vi "libssh2_session_disconnect_ex.vi"(7 "lang":string, 8 "error in (no error)":errorcluster, 9 "description":string, 10 "reason":i32, 11 "Session":T1) -> (0 "error out":errorcluster, 3 "return value":i32)   [LabVIEW 2013, in "libssh2.lvlib"]
uses:
  libssh2.lvlib
  Session Refnum.ctl
  libssh2.dll
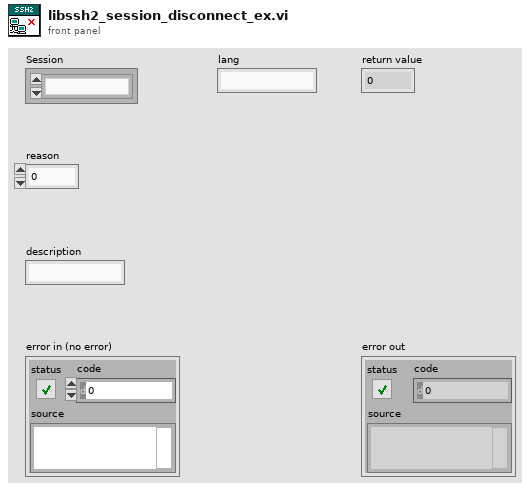
[diagram p1: front panel]
types:
  T1 = typedef "libssh2.lvlib/Session Refnum.ctl" = refnum<k1>
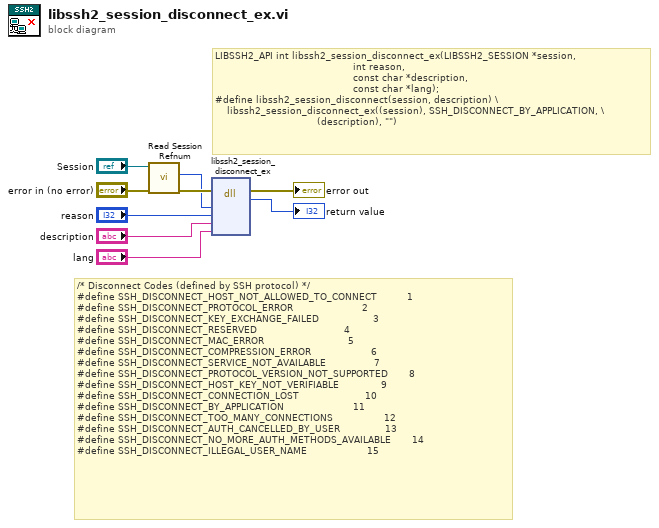
[diagram p0: block diagram]
diagram:
  # "/* Disconnect Codes (defined by SSH protocol) */\n#define SSH_DISCONNECT_HOST_NOT_ALLOWED_TO_CONNECT          1\n#define SSH_DISCONNECT_PROTOCOL_ERROR                       2\n#define SSH_DISCONNECT_KEY_EXCHANGE_FAILED                  3\n#define SSH_DISCONNECT_RESERVED                             4\n#define SSH_DISCONNECT_MAC_ERROR                            5\n#define SSH_DISCONNECT_COMPRESSION_ERROR                    6\n#define SSH_DISCONNECT_SERVICE_NOT_AVAILABLE                7\n#define SSH_DISCONNECT_PROTOCOL_VERSION_NOT_SUPPORTED       8\n#define SSH_DISCONNECT_HOST_KEY_NOT_VERIFIABLE              9\n#define SSH_DISCONNECT_CONNECTION_LOST                      10\n#define SSH_DISCONNECT_BY_APPLICATION                       11\n#define SSH_DISCONNECT_TOO_MANY_CONNECTIONS                 12\n#define SSH_DISCONNECT_AUTH_CANCELLED_BY_USER               13\n#define SSH_DISCONNECT_NO_MORE_AUTH_METHODS_AVAILABLE       14\n#define SSH_DISCONNECT_ILLEGAL_USER_NAME                    15"
  # "LIBSSH2_API int libssh2_session_disconnect_ex(LIBSSH2_SESSION *session,\n                                              int reason,\n                                              const char *description,\n                                              const char *lang);\n#define libssh2_session_disconnect(session, description) \\\n    libssh2_session_disconnect_ex((session), SSH_DISCONNECT_BY_APPLICATION, \\\n                                  (description), \"\")"
  n1 = call "Read Session Refnum.vi"("error in (no error)"="error in (no error)", "Session"="Session") -> ("error out"=w3:errorcluster, "LIBSSH2_SESSION*"=w1:u64)  [unwired: 8 in]
  n2 = dll-call lib="C:/Users/pasca/source/repos/libssh2-labview/libssh2**.*" fn="libssh2_session_disconnect_ex"(error in=w3, "session"=w1, "reason"="reason", "description"="description", "lang"="lang") -> (error out=→"error out":errorcluster, "return value"=→"return value":i32)  [unwired: 6 in, 1 out]
